vi "Periodic Tasks.vi"(8 "error in (no error)":errorcluster) -> ()   [LabVIEW 2020]
doc: "This VI runs in parallel to other tasks. It can contain as many user-defined periodic loops as you need. These can carry out PID or other sorts of timed response."
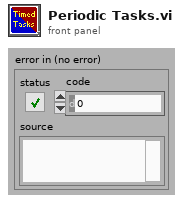
[diagram p1: front panel]
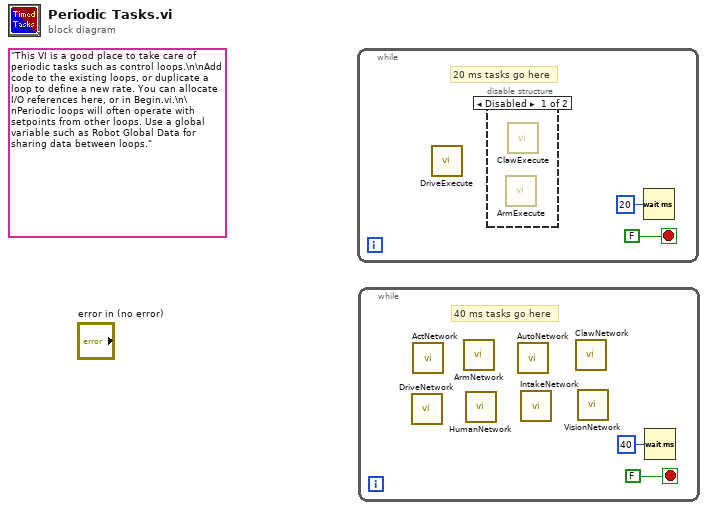
[diagram p0: block diagram]
diagram:
  (unwired) "This VI is a good place to take care of periodic tasks such as control loops.\n\nAdd code to the existing loops, or duplicate a loop to define a new rate. You can allocate I/O references here, or in Begin.vi.\n\nPeriodic loops will often operate with setpoints from other loops. Use a global variable such as Robot Global Data for sharing data between loops."
  n1 = while {
    stop <- FALSE stop-if-true
    # "20 ms tasks go here"
    n2 = call "DriveExecute.vi"() -> ()  [unwired: 11 in, 1 out]
    n3 = disable-structure shown="Disabled" {
      frame Disabled {
        n4 = call "ArmExecute.vi"() -> ()  [unwired: 12 in]
        n5 = call "ClawExecute.vi"() -> ()  [unwired: 12 in]
      }
      frame Enabled {
      }
    }
    n6 = Wait (ms)(milliseconds to wait=u32 20) -> ()  [unwired: 1 out]
  }
  n7 = while {
    stop <- FALSE stop-if-true
    # "40 ms tasks go here"
    n8 = call "DriveNetwork.vi"() -> ()  [unwired: 11 in, 1 out]
    n9 = call "ActNetwork.vi"() -> ()  [unwired: 11 in, 1 out]
    n10 = call "ArmNetwork.vi"() -> ()  [unwired: 11 in, 1 out]
    n11 = call "HumanNetwork.vi"() -> ()  [unwired: 11 in, 1 out]
    n12 = call "AutoNetwork.vi"() -> ()  [unwired: 11 in, 1 out]
    n13 = call "IntakeNetwork.vi"() -> ()  [unwired: 11 in, 1 out]
    n14 = call "ClawNetwork.vi"() -> ()  [unwired: 11 in, 1 out]
    n15 = call "VisionNetwork.vi"() -> ()  [unwired: 11 in, 1 out]
    n16 = Wait (ms)(milliseconds to wait=u32 40) -> ()  [unwired: 1 out]
  }
